vi "Control Value Update (Double).vi"(0 "Software Value":dbl, 5 "Hardware Value":dbl) -> (14 "New Software Value":dbl, 15 "Update Software":bool, 18 "New Hardware Value":dbl, 19 "Update Hardware":bool)   [LabVIEW 2011]
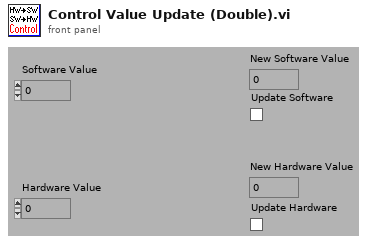
[diagram p1: front panel]
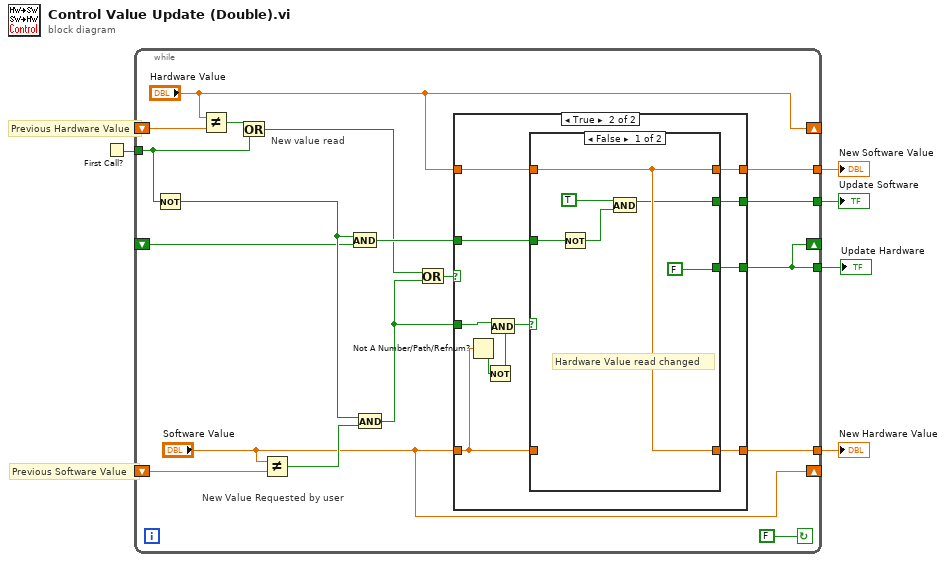
[diagram p0: block diagram]
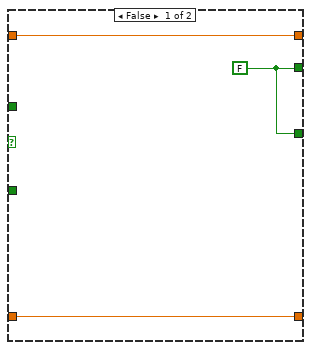
[diagram p2: hidden frame]
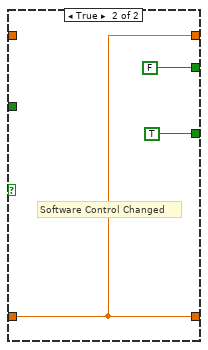
[diagram p3: hidden frame]
diagram:
  # "Previous Software Value"
  # "Previous Hardware Value"
  n1 = First Call?() -> (First Call?: T/F=w3:bool)
  n2 = while {
    tunnel: w3 -> [w22]
    shift-left: _ -> [w20]
    shift-right: ["Hardware Value"] -> _
    shift-right: ["Software Value"] -> _
    shift-left: _ -> [w19]
    tunnel: [w17] -> w5
    tunnel: [w14] -> w4
    shift-right: [w14] -> _
    shift-left: _ -> [w12]
    tunnel: [w9] -> w2
    tunnel: [w7] -> w1
    stop <- FALSE continue-if-true
    # "New Value Requested by user"
    # "New value read"
    n3 = Not(x=w22) -> (.not. x?=w13:bool)
    n4 = Not Equal?(x="Hardware Value", y=w20) -> (x != y?=w23:bool)
    n5 = Or(x=w23, y=w22) -> (x .or. y?=w6:bool)
    n6 = Not Equal?(x="Software Value", y=w19) -> (x != y?=w21:bool)
    n7 = And(x=w13, y=w12) -> (x .and. y?=w11:bool)
    n8 = And(x=w13, y=w21) -> (x .and. y?=w15:bool)
    n9 = Or(x=w6, y=w15) -> (x .or. y?=w18:bool)
    n10 = case shown="True" w18 {
      tunnel: "Hardware Value" -> [w26 w37]
      tunnel: [w25 w36] -> w17
      tunnel: [w25 w35] -> w14
      tunnel: [w26 w34] -> w9
      tunnel: [w24 w33] -> w7
      tunnel: "Software Value" -> [w24 w31]
      tunnel: w15 -> [_ w29]
      tunnel: w11 -> [_ w32]
      frame False {
        w25 = FALSE
      }
      frame True {
        n11 = Not A Number/Path/Refnum?(number/path/refnum=w31) -> (NaN/Path/Refnum?=w28:bool)
        n12 = Not(x=w28) -> (.not. x?=w27:bool)
        n13 = And(x=w29, y=w27) -> (x .and. y?=w30:bool)
        n14 = case shown="False" w30 {
          tunnel: w37 -> [w43 _]
          tunnel: [w38 FALSE] -> w36
          tunnel: [FALSE TRUE] -> w35
          tunnel: [w43 w45] -> w34
          tunnel: [w43 w45] -> w33
          tunnel: w31 -> [_ w45]
          tunnel: w32 -> [w41 _]
          frame False {
            # "Hardware Value read changed"
            n15 = Not(x=w41) -> (.not. x?=w39:bool)
            n16 = And(x=TRUE, y=w39) -> (x .and. y?=w38:bool)
          }
          frame True {
            # "Software Control Changed"
          }
        }
      }
    }
  }
  "New Software Value" <- w2
  "Update Software" <- w5
  "Update Hardware" <- w4
  "New Hardware Value" <- w1
